vi "Profile Y Value.vi"() -> ()   [LabVIEW 2010]
panel:
  in  "ramp Rate":string[](array[string])
  in  "AutoStart":string[](array[string])
  in  "Soak":string[](array[string])
  in  "Ramp Time":string[](array[string])
  out "Message Out":string[][](array[string])
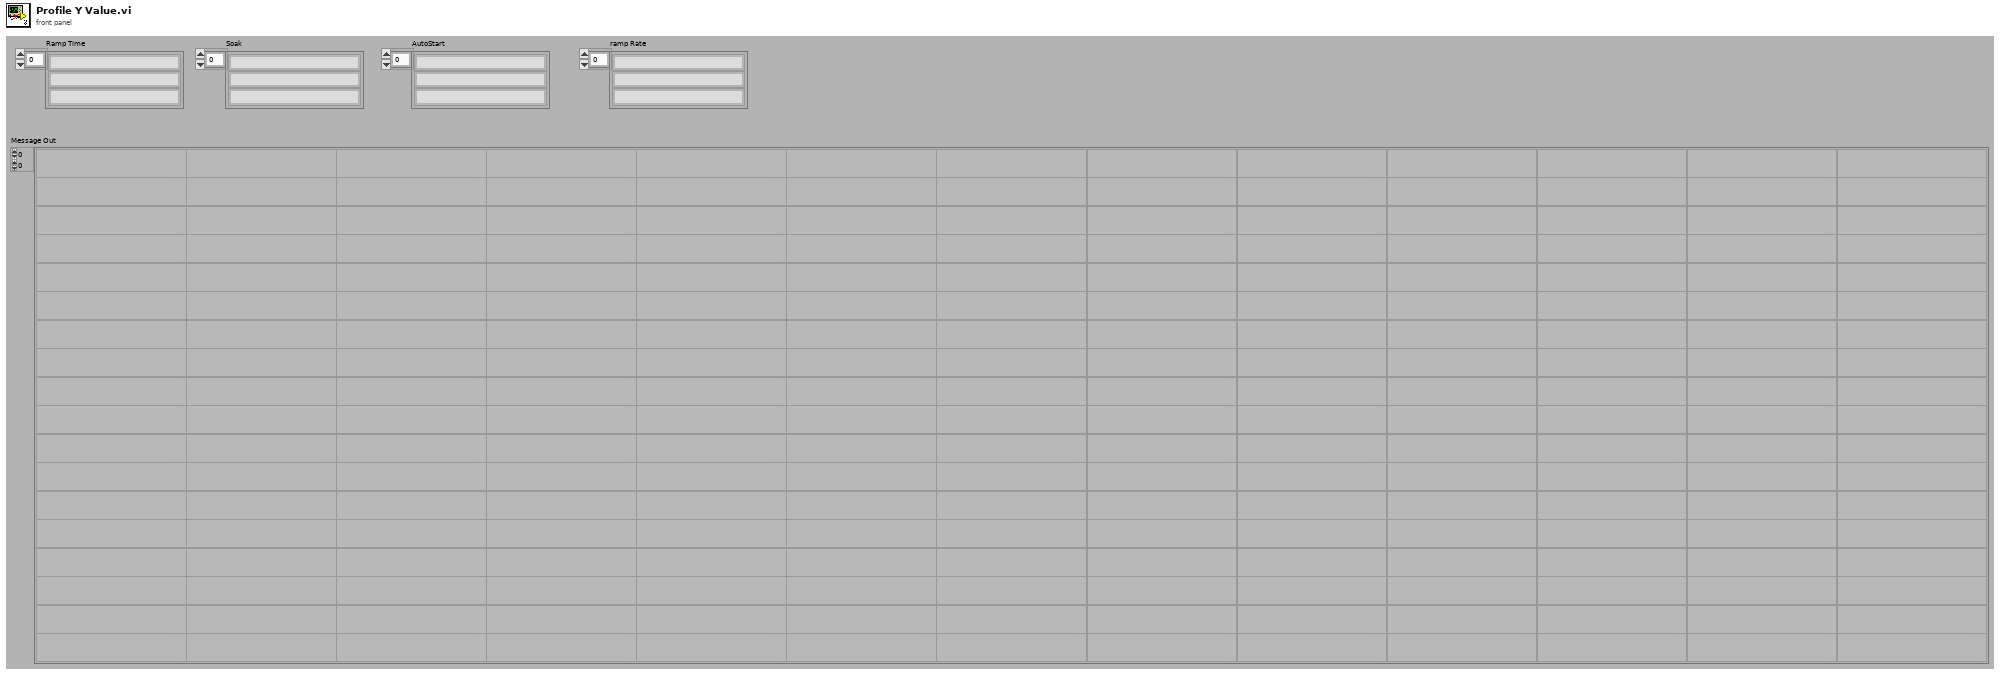
[diagram p1: front panel]
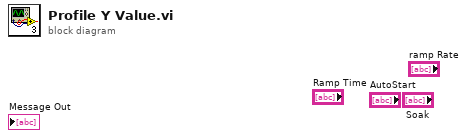
[diagram p0: block diagram]
diagram:
